vi "SawScan(Two axis + ISS option).vi"() -> ()   [LabVIEW 2012]
uses:
  Madlib.dll
panel:
  out "X Position (um)":dbl(graph)
  in  "X DELAY (ms)":u32=10
  in  "Y DELAY (ms)":u32=30
  out "Y Position (um)":dbl(graph)
  in  "Y Samples":u16=100 min=1 step=1
  in  "Y End  (um)":dbl=80.0 min=0.0 max=100.0 step=0.001 format="%.4f"
  in  "Y Start  (um)":dbl=20.0 min=0.0 max=100.0 step=0.5 format="%.3f"
  in  "X Samples":u16=100 min=1 step=1
  in  "X Start  (um)":dbl=20.0 min=0.0 max=100.0 step=0.5 format="%.3f"
  in  "X End  (um)":dbl=80.0 min=0.0 max=100.0 step=0.001 format="%.4f"
  # "This implements a Sawscan in X and Y and generates the proper clocks for a SPC board using \nthe Image Scan Sync (ISS) option."
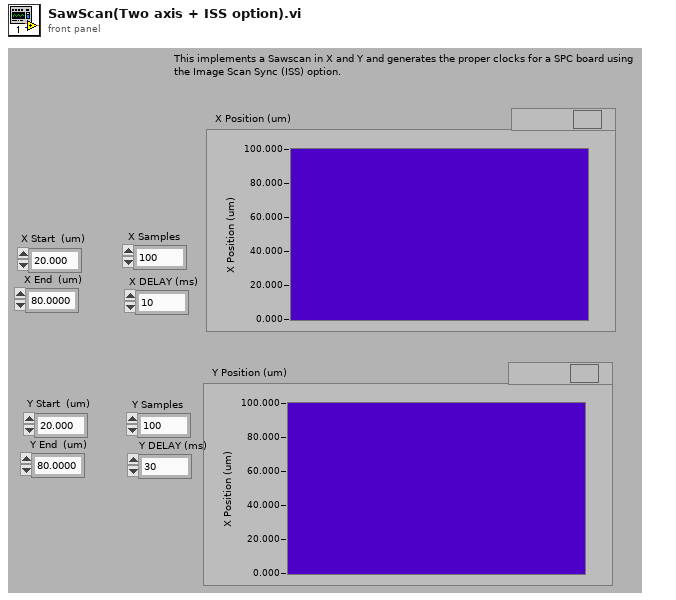
[diagram p1: front panel]
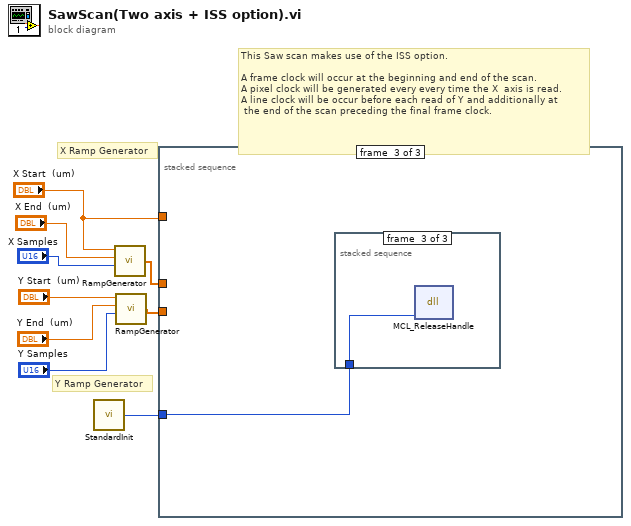
[diagram p0: block diagram]
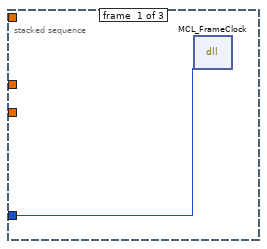
[diagram p2: hidden frame]
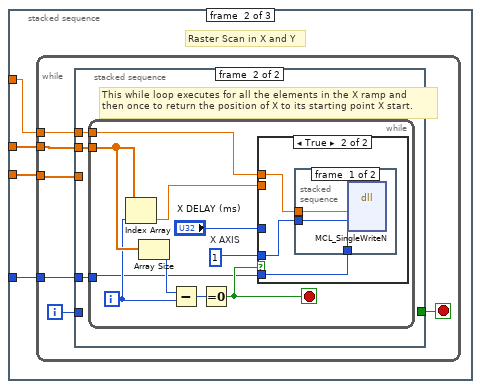
[diagram p3: hidden frame]
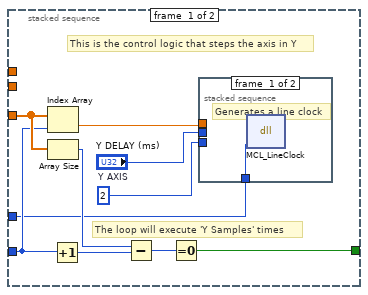
[diagram p4: hidden frame]
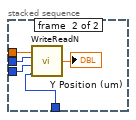
[diagram p5: hidden frame]
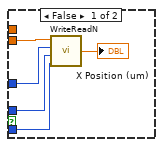
[diagram p6: hidden frame]
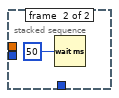
[diagram p7: hidden frame]
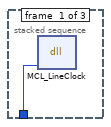
[diagram p8: hidden frame]
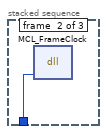
[diagram p9: hidden frame]
diagram:
  # "This Saw scan makes use of the ISS option. \n\nA frame clock will occur at the beginning and end of the scan.\nA pixel clock will be generated every every time the X  axis is read.\nA line clock will be occur before each read of Y and additionally at\n the end of the scan preceding the final frame clock."
  # "X Ramp Generator"
  # "Y Ramp Generator"
  n1 = call "StandardInit.vi"() -> ("Outgoing Handle"=w1:i32)  [unwired: 1 in]
  n2 = call "RampGenerator.vi"("Number of Positions"="X Samples", "End  (um)"="X End  (um)", "Start  (um)"="X Start  (um)") -> ("Array"=w9:dbl[])  [unwired: 1 in]
  n3 = call "RampGenerator.vi"("Number of Positions"="Y Samples", "End  (um)"="Y End  (um)", "Start  (um)"="Y Start  (um)") -> ("Array"=w8:dbl[])  [unwired: 1 in]
  n4 = stacked-sequence {
    tunnel: w9 -> [_ w13 _]
    tunnel: w8 -> [_ w14 _]
    tunnel: "X Start  (um)" -> [_ w12 _]
    tunnel: w1 -> [w10 w11 w62]
    frame #0 {
      n5 = dll-call lib="C:/Users/Labview/Desktop/SRR/Madlib_x64/Labview Examples/MADLib.dll" fn="MCL_FrameClock" label="Frame Clock"("handle"=w10) -> ()  [unwired: 5 in, 2 out]
    }
    frame #1 {
      # "Raster Scan in X and Y"
      n6 = while {
        tunnel: w14 -> [w20]
        tunnel: w12 -> [w17]
        tunnel: w13 -> [w16]
        tunnel: w11 -> [w15]
        i -> [w18]
        stop <- w19 stop-if-true
        # "X Ramp Generator"
        n7 = stacked-sequence {
          tunnel: w20 -> [w30 _]
          tunnel: [w28 _] -> w19
          tunnel: w18 -> [w24 _]
          tunnel: w16 -> [_ w39]
          tunnel: w17 -> [_ w38]
          tunnel: w15 -> [w21 w37]
          frame #0 {
            w25 = 2  # Y AXIS
            # "The loop will execute 'Y Samples' times"
            # "This is the control logic that steps the axis in Y"
            n8 = Index Array(array=w30, index=w24) -> (element=w22:dbl)
            n9 = Array Size(array=w30) -> (size(s)=w27:i32)
            n10 = Increment(x=w24) -> (x+1=w23:i32)
            n11 = Subtract(x=w27, y=w23) -> (x-y=w29:i32)
            n12 = Equal To 0?(x=w29) -> (x = 0?=w28:bool)
            n13 = stacked-sequence {
              tunnel: w22 -> [_ w36]
              tunnel: "Y DELAY (ms)" -> [_ w35]
              tunnel: w25 -> [_ w34]
              tunnel: w21 -> [w31 w32]
              frame #0 {
                # "Generates a line clock"
                n14 = dll-call lib="C:/Users/Labview/Desktop/SRR/Madlib_x64/Labview Examples/MADLib.dll" fn="MCL_LineClock"("handle"=w31) -> ()  [unwired: 5 in, 2 out]
              }
              frame #1 {
                n15 = call "WriteReadN.vi"("Handle"=w32, "Axis"=w34, "Delay (ms)"=w35, "Move to (um)"=w36) -> ("Current Position (um)"=→"Y Position (um)":dbl)
              }
            }
          }
          frame #1 {
            # "This while loop executes for all the elements in the X ramp and \nthen once to return the position of X to its starting point X start."
            n16 = while {
              tunnel: w39 -> [w47]
              tunnel: w38 -> [w42]
              tunnel: w37 -> [w40]
              i -> [w45]
              stop <- w46 stop-if-true
              w43 = 1  # X AXIS
              n17 = Index Array(array=w47, index=w45) -> (element=w41:dbl)
              n18 = Array Size(array=w47) -> (size(s)=w48:i32)
              n19 = Subtract(x=w48, y=w45) -> (x-y=w49:i32)
              n20 = Equal To 0?(x=w49) -> (x = 0?=w46:bool)
              n21 = case shown="True" w46 {
                tunnel: w41 -> [w53 _]
                tunnel: "X DELAY (ms)" -> [w52 _]
                tunnel: w43 -> [w51 w57]
                tunnel: w42 -> [_ w56]
                tunnel: w40 -> [w50 w55]
                frame False {
                  n22 = call "WriteReadN.vi"("Handle"=w50, "Axis"=w51, "Delay (ms)"=w52, "Move to (um)"=w53) -> ("Current Position (um)"=→"X Position (um)":dbl)
                }
                frame True {
                  # "X AXIS SCAN"
                  n23 = stacked-sequence {
                    tunnel: w57 -> [w60 _]
                    tunnel: w56 -> [w59 _]
                    tunnel: w55 -> [w58 _]
                    frame #0 {
                      n24 = dll-call lib="C:/Users/Labview/Desktop/SRR/Madlib_x64/Labview Examples/MADLib.dll" fn="MCL_SingleWriteN"("position"=w59, "axis"=w60, "handle"=w58) -> ()  [unwired: 7 in, 2 out]
                    }
                    frame #1 {
                      n25 = Wait (ms)(milliseconds to wait=50) -> ()  [unwired: 1 out]
                    }
                  }
                }
              }
            }
          }
        }
      }
    }
    frame #2 {
      # "End of Frame Clock"
      n26 = stacked-sequence {
        tunnel: w62 -> [w63 w64 w65]
        frame #0 {
          n27 = dll-call lib="C:/Users/Labview/Desktop/SRR/Madlib_x64/Labview Examples/MADLib.dll" fn="MCL_LineClock" label="Line Clock"("handle"=w63) -> ()  [unwired: 5 in, 2 out]
        }
        frame #1 {
          n28 = dll-call lib="C:/Users/Labview/Desktop/SRR/Madlib_x64/Labview Examples/MADLib.dll" fn="MCL_FrameClock" label="Frame Clock"("handle"=w64) -> ()  [unwired: 5 in, 2 out]
        }
        frame #2 {
          n29 = dll-call lib="C:/Users/Labview/Desktop/SRR/Madlib_x64/Labview Examples/MADLib.dll" fn="MCL_ReleaseHandle"("handle"=w65) -> ()  [unwired: 5 in, 2 out]
        }
      }
    }
  }
